vi "Read conditional terminal.vi"(9 "LoopTunnel in":refnum<class "LoopTunnel.lvclass">) -> (3 "LoopTunnel out":refnum<class "LoopTunnel.lvclass">, 4 "Terminal.lvclass":refnum<class "Terminal.lvclass">)   [LabVIEW 2014, in "LoopTunnel.lvclass"]
uses:
  LoopTunnel.lvclass
  Terminal/Terminal.lvclass
  LoopTunnel.lvclass/LoopTunnel.ctl
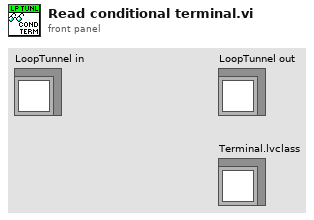
[diagram p1: front panel]
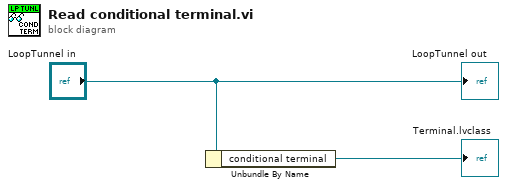
[diagram p0: block diagram]
diagram:
  n1 = Unbundle By Name("LoopTunnel in") -> ("conditional terminal"=→"Terminal.lvclass":refnum<class "Terminal.lvclass">)
  "LoopTunnel out" <- "LoopTunnel in"
